vi "SubVI – teaching (invatare) – Validation (validare).vi"(2 "Nr Val Validare":dbl, 3 "Nr Val Esantion":dbl, 4 "H minim m":dbl, 5 "H maxim m":dbl, 6 "Masa Minima KG":dbl, 7 "Masa Maxima KG":dbl) -> (0 "RNLAB4TestValidation PATH":path, 1 "RNLAB4TestTeaching PATH":path)   [LabVIEW 2024]
uses:
  <vilib>/National Instruments/NI Super Simple Neural Networks/Types/Teaching Vector.ctl
  <vilib>/National Instruments/NI Super Simple Neural Networks/Types/1D Array.ctl
  <vilib>/National Instruments/NI Super Simple Neural Networks/Neural Network.lvclass
panel:
  in  "Teaching Vector 2":T1
  in  "Teaching Vector":T1
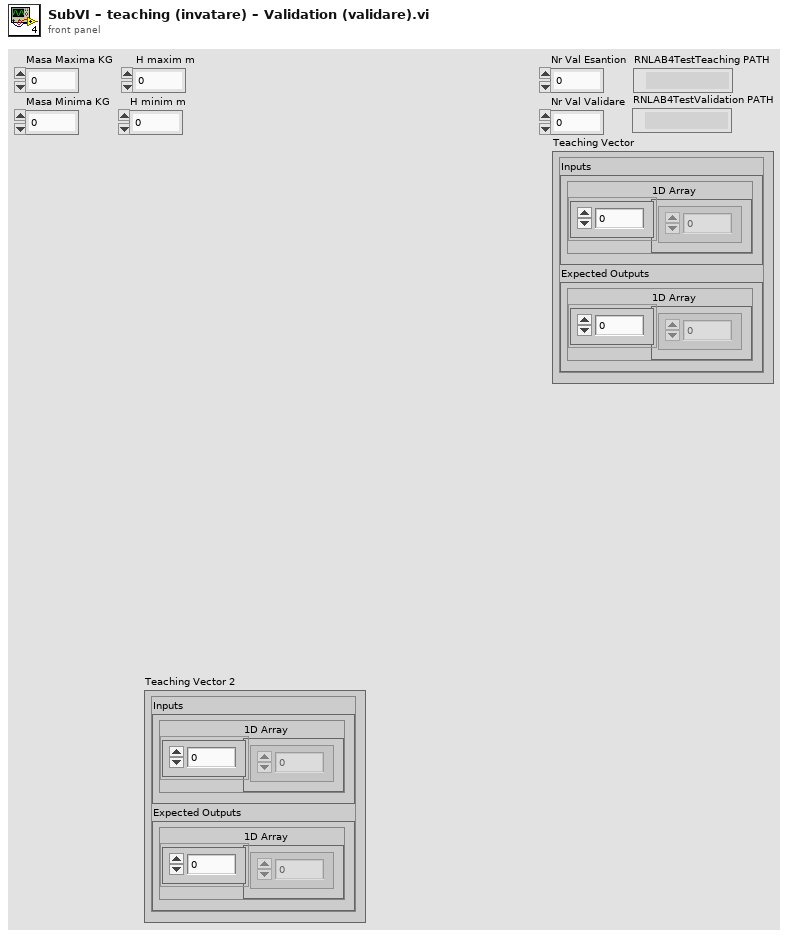
[diagram p1: front panel]
types:
  T1 = typedef "Neural Network.lvclass/Teaching Vector.ctl" = cluster{"Inputs":T2, "Expected Outputs":T2}
  T2 = typedef "Neural Network.lvclass/1D Array.ctl" = cluster{"1D Array":dbl[]}
  T3 = enum16{"open", "replace", "create", "open or create", "replace or create", "replace or create with confirmation"}
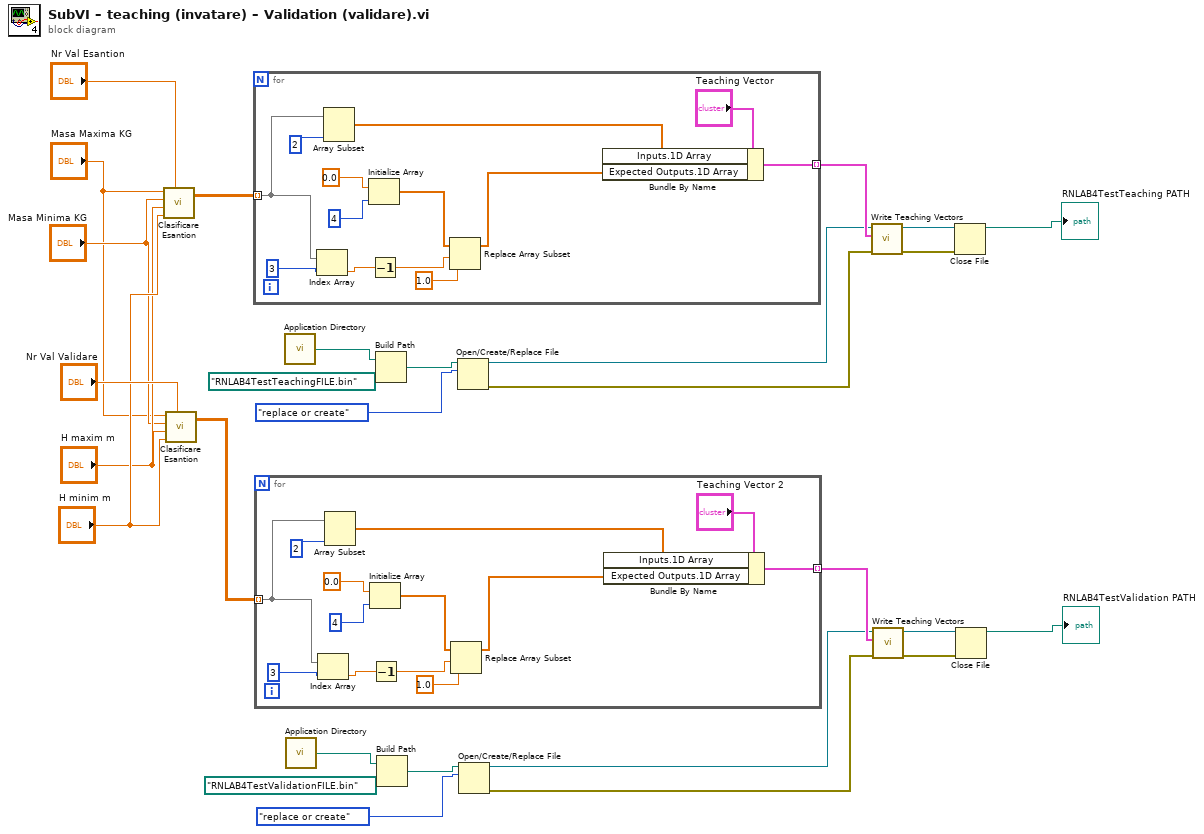
[diagram p0: block diagram]
diagram:
  n1 = call "Clasificare Esantion.vi"("Masa Maxima KG"="Masa Maxima KG", "Masa Minima KG"="Masa Minima KG", "H maxim m"="H maxim m", "H minim m"="H minim m", "Nr Val Esantion"="Nr Val Esantion") -> ("Esantion Clasificat"=w22:dbl[][])  [unwired: 1 out]
  n2 = call "Clasificare Esantion.vi"("Masa Maxima KG"="Masa Maxima KG", "Masa Minima KG"="Masa Minima KG", "H maxim m"="H maxim m", "H minim m"="H minim m", "Nr Val Esantion"="Nr Val Validare") -> ("Esantion Clasificat"=w1:dbl[][])  [unwired: 1 out]
  n3 = for {
    tunnel: w22 -> [w39] mode=indexing
    tunnel: [w29] -> w21 mode=indexing
    n4 = Index Array(array=w39, index=3) -> (element=w35:dbl)
    n5 = Array Subset(array=w39, length=2) -> (w31:dbl[])  [unwired: 1 in]
    n6 = Initialize Array(0.0 ("element"), 4 ("dimension size")) -> (w36:dbl[])
    n7 = Decrement(x=w35) -> (x-1=w34:dbl)
    n8 = Replace Array Subset(array=w36, new element=1.0 ("new element/subarray"), index=w34) -> (w32:dbl[])
    n9 = Bundle By Name(cluster="Teaching Vector", "Inputs.1D Array"=w31, "Expected Outputs.1D Array"=w32) -> (w29:T1)
  }
  n10 = for {
    tunnel: w1 -> [w52] mode=indexing
    tunnel: [w42] -> w11 mode=indexing
    n11 = Index Array(array=w52, index=3) -> (element=w48:dbl)
    n12 = Array Subset(array=w52, length=2) -> (w44:dbl[])  [unwired: 1 in]
    n13 = Initialize Array(0.0 ("element"), 4 ("dimension size")) -> (w49:dbl[])
    n14 = Decrement(x=w48) -> (x-1=w47:dbl)
    n15 = Replace Array Subset(array=w49, new element=1.0 ("new element/subarray"), index=w47) -> (w45:dbl[])
    n16 = Bundle By Name(cluster="Teaching Vector 2", "Inputs.1D Array"=w44, "Expected Outputs.1D Array"=w45) -> (w42:T1)
  }
  n17 = call <vilib>:"Application Directory.vi"() -> ("Application Directory"=w18:path)
  n18 = call <vilib>:"Application Directory.vi"() -> ("Application Directory"=w8:path)
  n19 = Build Path(base path=w18, name or relative path=path "RNLAB4TestTeachingFILE.bin") -> (appended path=w17:path)
  n20 = Build Path(base path=w8, name or relative path=path "RNLAB4TestValidationFILE.bin") -> (appended path=w7:path)
  n21 = Open/Create/Replace File(file path (use dialog)=w17, operation (0:open)=T3."replace or create") -> (refnum out=w14:refnum<file>, error out=w13:errorcluster)  [unwired: 4 in, 1 out]
  n22 = Open/Create/Replace File(file path (use dialog)=w7, operation (0:open)=T3."replace or create") -> (refnum out=w4:refnum<file>, error out=w3:errorcluster)  [unwired: 4 in, 1 out]
  n23 = call <vilib>:"Write Teaching Vectors.vi"("Error In"=w13, "Teaching Vectors"=w21, "Teaching File Ref In"=w14) -> ("Error Out"=w19:errorcluster, "Teaching File Ref Out"=w20:refnum<file>)  [unwired: 7 in]
  n24 = call <vilib>:"Write Teaching Vectors.vi"("Error In"=w3, "Teaching Vectors"=w11, "Teaching File Ref In"=w4) -> ("Error Out"=w9:errorcluster, "Teaching File Ref Out"=w10:refnum<file>)  [unwired: 7 in]
  n25 = Close File(refnum=w20, error in=w19) -> (path=→"RNLAB4TestTeaching PATH":path)  [unwired: 1 out]
  n26 = Close File(refnum=w10, error in=w9) -> (path=→"RNLAB4TestValidation PATH":path)  [unwired: 1 out]
